vi "Integral x(t) PtByPt Vector.vi"(7 "initialize":bool, 8 "dt":dbl=1.0 format="%0.2f", 10 "Initial condition":dbl[](array[numeric]) format="%0.2f", 11 "x":dbl[](array[numeric]) format="%0.2f") -> (3 "Integral x(t)":dbl[](array[numeric]) format="%0.2f")   [LabVIEW 2012]
panel:
  # "Vector version of point-by-point simpson's rule integration.  If IC is empty (or not supplied)  then use 0 as IC.   Also, this version handles IC correctly, unlike the NI version."
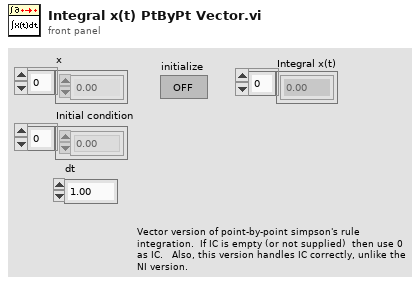
[diagram p1: front panel]
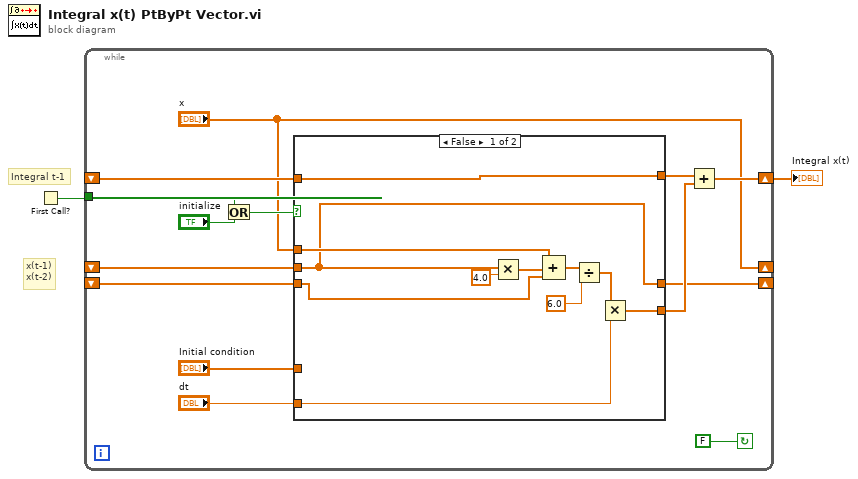
[diagram p0: block diagram]
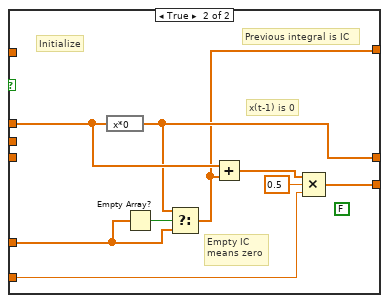
[diagram p2: hidden frame]
diagram:
  # "Integral t-1"
  # "x(t-1)\nx(t-2)"
  n1 = First Call?() -> (First Call?: T/F=w2:bool)
  n2 = while {
    shift-left: _ -> [w9]
    shift-right: [w6] -> w1
    tunnel: w2 -> [w14]
    shift-left: _ -> [w11]
    shift-right: ["x"] -> _
    shift-right: [w3] -> _
    shift-left: _ -> [w4]
    stop <- FALSE continue-if-true
    n3 = Or(x=w14, y="initialize") -> (x .or. y?=w13:bool)
    n4 = case shown="False" w13 {
      tunnel: "dt" -> [w27 w34]
      tunnel: "x" -> [w25 w32]
      tunnel: "Initial condition" -> [_ w31]
      tunnel: [w26 w36] -> w7
      tunnel: w11 -> [w21 _]
      tunnel: w4 -> [w22 _]
      tunnel: [w24 w28] -> w8
      tunnel: w9 -> [w24 _]
      tunnel: [w21 w30] -> w3
      frame False {
        n5 = Multiply(x=w21, y=4.0) -> (x*y=w19:dbl[])
        n6 = Compound Arithmetic op=ADD(w25, w19, w22) -> (w18:dbl[])
        n7 = Divide(x=w18, y=6.0) -> (x/y=w23:dbl[])
        n8 = Multiply(x=w23, y=w27) -> (x*y=w26:dbl[])
      }
      frame True {
        (unwired) FALSE ("Boolean")
        # "Previous integral is IC"
        # "x(t-1) is 0"
        # "Empty IC\nmeans zero"
        # "Initialize"
        n9 = expression code="x*0"(w32) -> (w30:dbl[])
        n10 = Empty Array?(array=w31) -> (empty?=w33:bool)
        n11 = Select(t=w30, s=w33, f=w31) -> (s? t:f=w28:dbl[])
        n12 = Add(x=w32, y=w28) -> (x+y=w29:dbl[])
        n13 = Compound Arithmetic op=MULTIPLY(w29, 0.5 ("Input"), w34) -> (w36:dbl[])
      }
    }
    n14 = Add(x=w8, y=w7) -> (x+y=w6:dbl[])
  }
  "Integral x(t)" <- w1
